vi "DB insert.vi"(7 "table Name":string, 8 "error in (no error)":errorcluster, 9 "Column Name":string[](array[string]), 10 "Column Values":string[][](array[string]), 11 "Db Reference":refnum<k24>) -> (0 "error out":errorcluster, 3 "Db Reference":refnum<k24>)   [LabVIEW 2020]
uses:
  D:/Labview/Auto Run Screen/Source Code/Database/Support/dbquery.dll
  Support/dbquery.dll
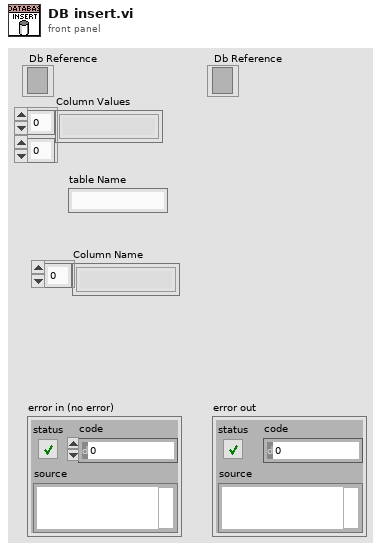
[diagram p1: front panel]
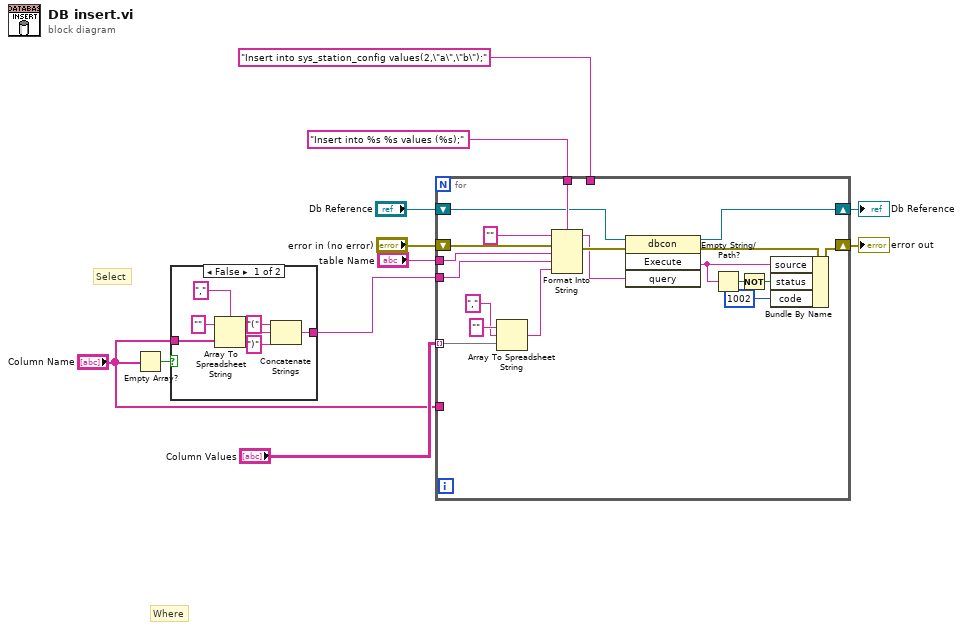
[diagram p0: block diagram]
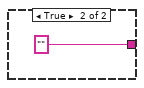
[diagram p2: hidden frame]
diagram:
  # "Where"
  # "Select"
  n1 = Empty Array?(array="Column Name") -> (empty?=w7:bool)
  n2 = case shown="False" w7 {
    tunnel: [w14 ""] -> w6
    tunnel: "Column Name" -> [w18 _]
    frame False {
      n3 = Array To Spreadsheet String(delimiter (Tab)=",", array=w18, 3:"" ("format string")) -> (spreadsheet string=w15:string)
      n4 = Concatenate Strings("(" ("string"), w15, ")" ("string")) -> (w14:string)
    }
    frame True {
    }
  }
  n5 = for {
    tunnel: "Insert into %s %s values (%s);" ("format string") -> [w38]
    tunnel: "table Name" -> [w32]
    tunnel: w6 -> [w31]
    shift-right: [w27] -> w11
    shift-left: "Db Reference" -> [w26]
    shift-right: [w24] -> w1
    shift-left: "error in (no error)" -> [w36]
    tunnel: "Column Values" -> [w30] mode=indexing
    tunnel: "Column Name" -> [_]
    tunnel: "Insert into sys_station_config values(2,\"a\",\"b\");" ("format string") -> [_]
    n6 = Array To Spreadsheet String(delimiter (Tab)=",", array=w30, 3:"" ("format string")) -> (spreadsheet string=w33:string)
    n7 = Format Into String(format string=w38, initial string="", error in=w36, w32, w31, w33) -> (resulting string=w25:string, error out=w29:errorcluster)
    n8 = invoke class="dbcon" method="Execute"(reference=w26, error in=w29, "query"=w25) -> (reference out=w27:refnum<k24>, error out=w28:errorcluster, "Execute"=w22:string)  [unwired: 1 in, 1 out]
    n9 = Empty String/Path?(string/path=w22) -> (empty?=w21:bool)
    n10 = Not(x=w21) -> (.not. x?=w20:bool)
    n11 = Bundle By Name(cluster=w28, "source"=w22, "status"=w20, "code"=1002) -> (w24:errorcluster)
  }
  "error out" <- w1
  "Db Reference" <- w11
